vi "get initial information.vi"(8 "error in (no error)":errorcluster, 10 "channel":u16, 11 "CCDCamera in":refnum<class "Real Camera.lvclass">) -> (0 "error out":errorcluster, 2 "ccd on/off":bool, 3 "CCDCamera out":refnum<class "Real Camera.lvclass">)   [LabVIEW 2018, in "Real Camera.lvclass"]
uses:
  Real Camera.lvclass
  C:/Users/Denis/Desktop/S4ACS/S4ACS/Simulated_CCD_Camera/Simulated Camera.lvclass
  Simulated_CCD_Camera/Simulated Camera.lvclass
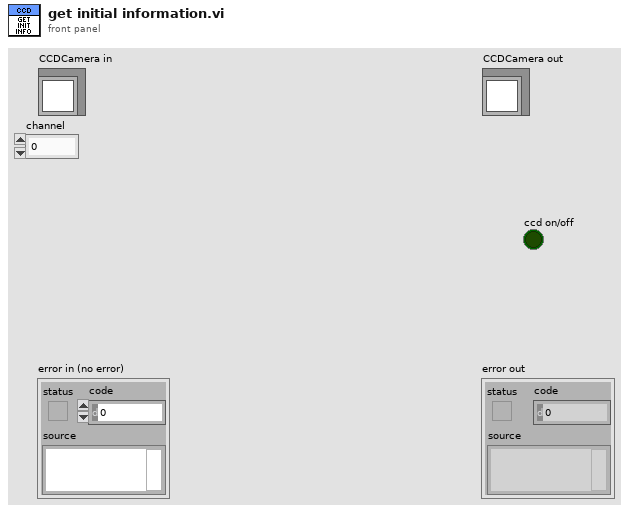
[diagram p1: front panel]
types:
  T1 = cluster{"CYCLES_DONE":u16, "LAST_IMAGE_NAME":string, "DISK_SPACE":u16, "FRAMES_DONE":u16, "CCD_STATUS":string, "CURRENT_TEMPERATURE":i16, "TEMPERATURE_STATUS":string, "FRAME_EXPOSURE_TIME":sgl, "ERROR":bool, "SERIAL_NUMBER":u16, "ACQUIRING":bool, "IMAGE_INDEX":u32, "SEQS_DONE":u16}
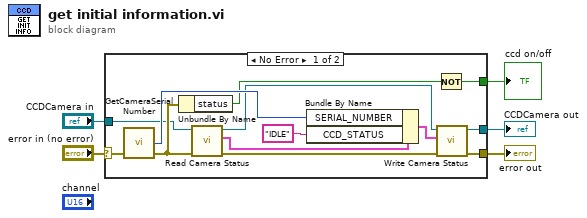
[diagram p0: block diagram]
diagram:
  n1 = case shown="No Error" "error in (no error)" {
    selector: "error in (no error)" -> [w10 w20]
    tunnel: "CCDCamera in" -> [w9 w19]
    tunnel: [w8 w19] -> w3
    tunnel: [w7 w20] -> w2
    tunnel: [w6 _] -> w1
    frame No Error {
      n2 = call <userlib>:"GetCameraSerialNumber.vi"("error in (no error)"=w10) -> ("error out"=w12:errorcluster, "number"=w17:i32)  [unwired: 2 in, 1 out]
      n3 = Unbundle By Name(w12) -> ("status"=w11:bool)
      n4 = call "Read Camera Status.vi"("error in (no error)"=w12, "CCDCamera in"=w9) -> ("error out"=w16:errorcluster, "Camera Status"=w14:T1, "CCDCamera out"=w15:refnum<class "Real Camera.lvclass">)  [unwired: 7 in]
      n5 = Bundle By Name(cluster=w14, "SERIAL_NUMBER"=w17, "CCD_STATUS"="IDLE" ("Camera Status.STATUS")) -> (w13:T1)
      n6 = Not(x=w11) -> (.not. x?=w6:bool)
      n7 = call "Write Camera Status.vi"("error in (no error)"=w16, "Camera Status"=w13, "CCDCamera in"=w15) -> ("error out"=w7:errorcluster, "CCDCamera out"=w8:refnum<class "Real Camera.lvclass">)  [unwired: 7 in]
    }
    frame Error {
    }
  }
  "error out" <- w2
  "CCDCamera out" <- w3
  "ccd on/off" <- w1
